vi "Pack Multiple 24xI16 to 32xI16.vi"(8 "Input Valid":bool, 11 "Input Data":i16[](array[numeric])=[0, 0, 0, 0, 0, 0, 0, 0, 0, 0, 0, 0, 0, 0, 0, 0, 0, 0, 0, 0, 0, 0, 0, 0]) -> (0 "Output Valid":bool, 3 "Output Data":i16[](array[numeric]))   [LabVIEW 2012]
doc: "<b> Latency = 2 Ticks </b>"
uses:
  <vilib>/rvi/FXPMathLib/basic elements/FxpDiscreteDelay/XNode/nifxpmath_DiscreteDelay.xnode
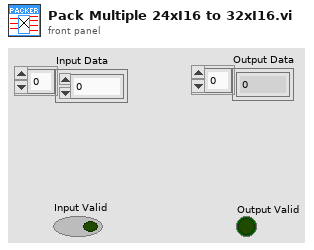
[diagram p1: front panel]
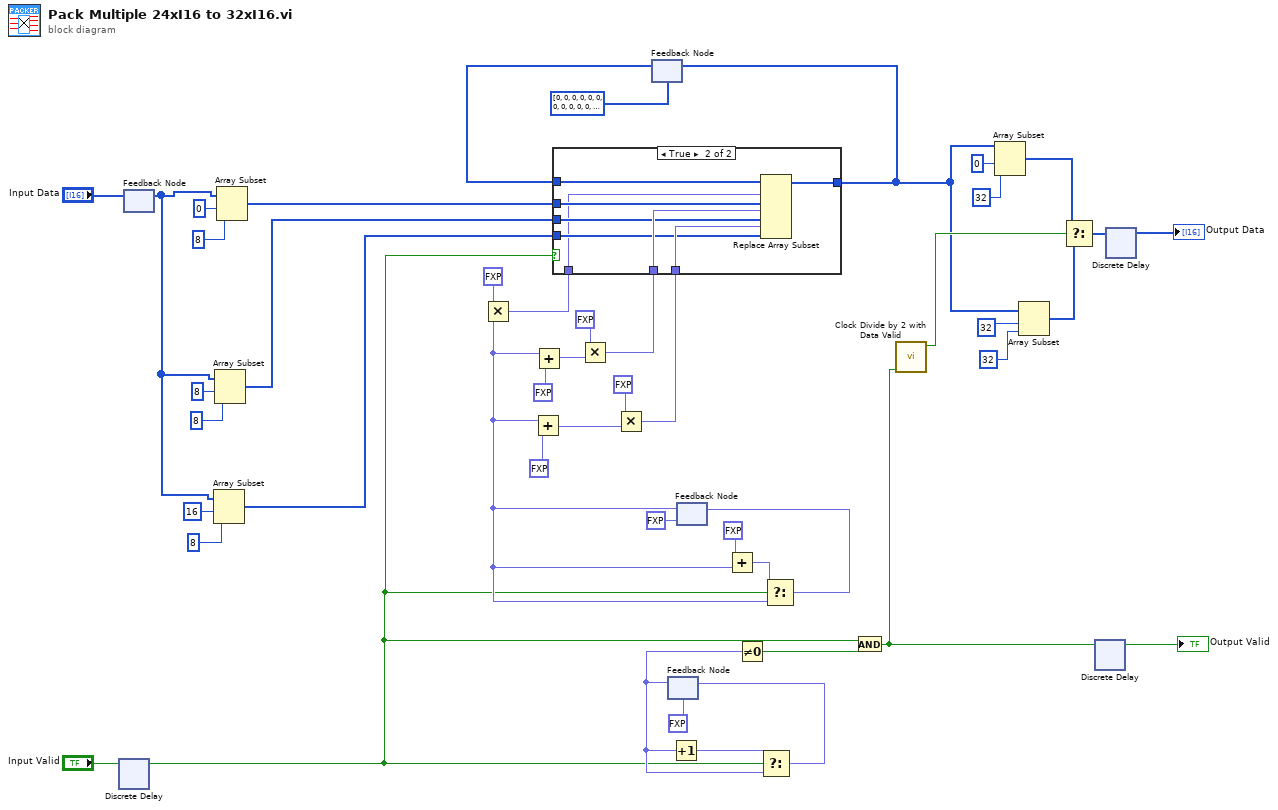
[diagram p0: block diagram]
diagram:
  n1 = xnode "Discrete Delay"("D"="Input Valid") -> ("Q"=w3:bool)
  n2 = feedback-in #1("Input Data") -> ()
  n3 = feedback #1() -> (w4:i16[])  [unwired: 1 in]
  n4 = Array Subset(array=w4, index=16, length=8) -> (w25:i16[])
  n5 = Array Subset(array=w4, index=8, length=8) -> (w28:i16[])
  n6 = Array Subset(array=w4, index=0, length=8) -> (w33:i16[])
  n7 = feedback #2(i16[] [0, 0, 0, 0, 0, 0, 0, 0, 0, 0, 0, 0, 0, 0, 0, 0, 0, 0, 0, 0, 0, 0, 0, 0, 0, 0, 0, 0, 0, 0, 0, 0, 0, 0, 0, 0, 0, 0, 0, 0, 0, 0, 0, 0, 0, 0, 0, 0, 0, 0, 0, 0, 0, 0, 0, 0, 0, 0, 0, 0, 0, 0, 0, 0]) -> (w46:i16[])
  n8 = feedback #3(fxp<+,2,2> 0.0) -> (w38:fxp<+,2,2>)
  n9 = Increment(x=w38) -> (x+1=w39:fxp<+,2,2>)
  n10 = feedback #4(fxp<+,3,3> 0.0) -> (w35:fxp<+,3,3>)
  n11 = Multiply(x=fxp<+,4,4> 8.0, y=w35) -> (x*y=w23:fxp<+,7,7>)
  n12 = Add(x=w35, y=fxp<+,3,3> 2.0) -> (x+y=w19:fxp<+,3,3>)
  n13 = Add(x=w35, y=fxp<+,3,3> 1.0) -> (x+y=w22:fxp<+,3,3>)
  n14 = Multiply(x=fxp<+,4,4> 8.0, y=w22) -> (x*y=w20:fxp<+,7,7>)
  n15 = Multiply(x=fxp<+,4,4> 8.0, y=w19) -> (x*y=w18:fxp<+,7,7>)
  n16 = case shown="True" w3 {
    tunnel: w46 -> [w48 w56]
    tunnel: w20 -> [_ w55]
    tunnel: w18 -> [_ w54]
    tunnel: [w48 w53] -> w5
    tunnel: w33 -> [_ w52]
    tunnel: w28 -> [_ w51]
    tunnel: w25 -> [_ w50]
    tunnel: w23 -> [_ w49]
    frame False {
    }
    frame True {
      n17 = Replace Array Subset(array=w56, new element #1=w52, index #1=w49, new element #2=w51, index #2=w55, new element #3=w50, index #3=w54) -> (w53:i16[])
    }
  }
  n18 = feedback-in #2(w5) -> ()
  n19 = Add(x=fxp<+,3,3> 3.0, y=w35) -> (x+y=w36:fxp<+,3,3>)
  n20 = Not Equal To 0?(x=w38) -> (x != 0?=w37:bool)
  n21 = Select(t=w39, s=w3, f=w38) -> (s? t:f=w40:fxp<+,2,2>)
  n22 = feedback-in #3(w40) -> ()
  n23 = Select(t=w36, s=w3, f=w35) -> (s? t:f=w15:fxp<+,3,3>)
  n24 = feedback-in #4(w15) -> ()
  n25 = And(x=w3, y=w37) -> (x .and. y?=w13:bool)
  n26 = call <userlib>:"Clock Divide by 2 with Data Valid.vi"("Data Valid"=w13) -> ("CLK/2"=w14:bool)  [unwired: 10 in]
  n27 = Array Subset(array=w5, index=0, length=32) -> (w8:i16[])
  n28 = Array Subset(array=w5, index=32, length=32) -> (w7:i16[])
  n29 = Select(t=w8, s=w14, f=w7) -> (s? t:f=w6:i16[])
  n30 = xnode "Discrete Delay"("D"=w13) -> ("Q"=→"Output Valid":bool)
  n31 = xnode "Discrete Delay"("D"=w6) -> ("Q"=→"Output Data":i16[])
